vi "OP70_Data.vi"() -> (0 "OP70_ASR":T1)   [LabVIEW 2020]
panel:
  out "error out":errorcluster
  in  "OP80_ASR_MAX_LOAD":dbl
  in  "ASR DISTANCE":dbl
  in  "ASR":dbl
  in  "[CT]":dbl
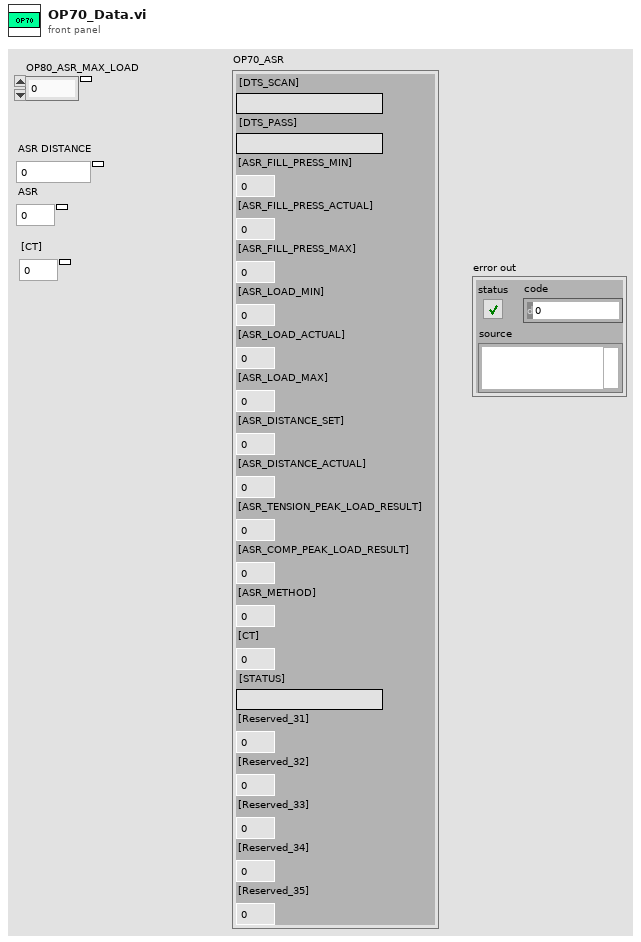
[diagram p1: front panel]
types:
  T1 = cluster{"[DTS_SCAN]":string, "[DTS_PASS]":string, "[ASR_FILL_PRESS_MIN]":dbl, "[ASR_FILL_PRESS_ACTUAL]":dbl, "[ASR_FILL_PRESS_MAX]":dbl, "[ASR_LOAD_MIN]":dbl, "[ASR_LOAD_ACTUAL]":dbl, "[ASR_LOAD_MAX]":dbl, "[ASR_DISTANCE_SET]":dbl, "[ASR_DISTANCE_ACTUAL]":dbl, "[ASR_TENSION_PEAK_LOAD_RESULT]":dbl, "[ASR_COMP_PEAK_LOAD_RESULT]":dbl, "[ASR_METHOD]":dbl, "[CT]":dbl, "[STATUS]":string, "[Reserved_31]":dbl, "[Reserved_32]":dbl, "[Reserved_33]":dbl, "[Reserved_34]":dbl, "[Reserved_35]":dbl}
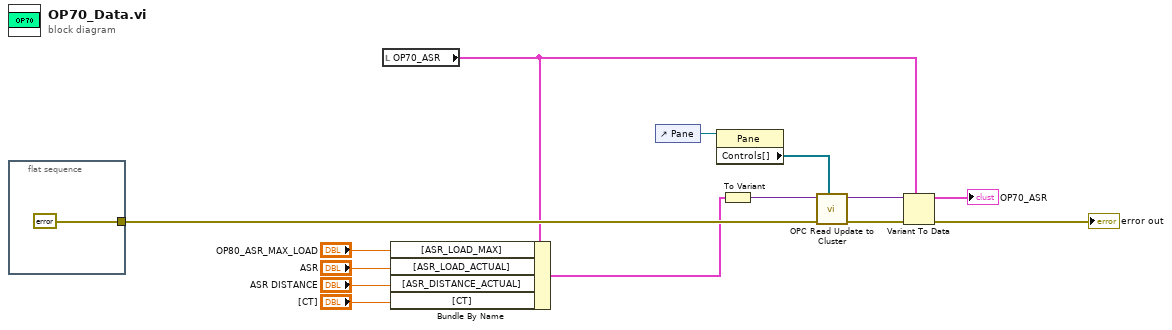
[diagram p0: block diagram]
diagram:
  n1 = flat-sequence {
    tunnel: [errorcluster {"status"=FALSE, "code"=0, "source"=""} ("error in (no error)")] -> w11
    frame #0 {
    }
  }
  n2 = local read "OP70_ASR"() -> (w7:T1)
  n3 = Bundle By Name(cluster=w7, "[ASR_LOAD_MAX]"="OP80_ASR_MAX_LOAD", "[ASR_LOAD_ACTUAL]"="ASR", "[ASR_DISTANCE_ACTUAL]"="ASR DISTANCE", "[CT]"="[CT]") -> (w6:T1)
  n4 = control-ref of="Pane"() -> (w10:refnum<vi>)
  n5 = property class="Pane"(reference=w10) -> ("Controls[]"=w9:refnum<vi>[])  [unwired: 1 in, 2 out]
  n6 = To Variant(anything=w6) -> (Variant=w12:variant)
  n7 = call "OPC Read Update to Cluster.vi"("Controls[]"=w9, "error in (no error)"=w11, "Variant in"=w12) -> ("error out"=w13:errorcluster, "Variant out"=w14:variant)  [unwired: 7 in]
  n8 = Variant To Data(error in=w13, type=w7, Variant=w14) -> (data=→"OP70_ASR":T1, error out=→"error out":errorcluster)
